vi "BNC555.Read Channel Parameters.vi"(0 "i ref in":refnum<vi>, 2 "Channel (1: Chan A)":i32(ring)=1 items=["System (To)", "Channel A", "Channel B", "Channel C", "Channel D", "Channel E", "Channel F", "Channel G", "Channel H"], 3 "Parameter":T1(ring), 5 "error in (no error)":errorcluster) -> (14 "i ref out":refnum<vi>, 19 "error out":errorcluster)   [LabVIEW 2014, in "BNC555.lvlib"]
doc: "This VI queries the connected channel state. The result is indicated as GUI element, parts are published as a dim service."
uses:
  BNC555.lvlib
  instr.lib/BNC555/BNC555 - Driver np.lvlib
  CSlibraries-extern/DimLVEvent/LVDimInterface/LVDimInterface.lvlib
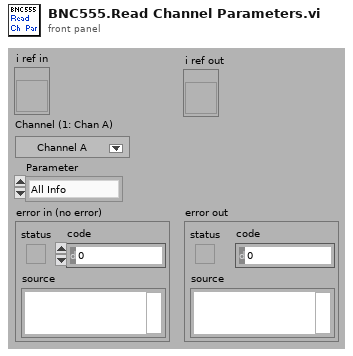
[diagram p1: front panel]
types:
  T1 = enum16{"All Info", "State (On/Off)", "Output Config", "Mode Config", "Pulse Config", "Gate Config"}
  T2 = typedef "BNC555.lvlib/BNC555.i attribute.ctl" = cluster{"Information":cluster{"VISA resource name":refnum<visa-resource-name>, "Baud Rate (1:9600)":u16}, "Channel Array":T3[], "System":T4, "GUI Refs":cluster{"Delete":refnum<vi>, "Information":refnum<vi>, "System":refnum<vi>, "Channel Array":refnum<vi>, "Device Error":refnum<vi>, "Instr Driver Revision":refnum<vi>, "Instr Firmware Revision":refnum<vi>, "Instr Option":refnum<vi>, "Self-Test Response":refnum<vi>}, "Service IDs Channelinfo":i32[], "Service ID T0 Mode":i32}
  T3 = typedef "BNC555 - Driver np.lvlib/BNC555 All Chan Parameters.ctl" = cluster{"Chan #":i32, "Chan State":bool, "Chan Delay":dbl, "Chan Width":dbl, "Chan Mode":enum16{"Normal", "Single", "Burst", "Divide by N"}, "Chan Burst #":u32, "Chan Divide #":u32, "Chan Pol Out":enum16{"Normal", "Complement", "Inverted"}, "Chan Level Out":enum16{"TTL", "Adjustable", "35 Volt"}, "Chan Lev Adjust":dbl, "Chan Gate Pol":enum16{"Normal", "Complement", "Inverted"}, "Chan Gate State":bool}
  T4 = typedef "BNC555 - Driver np.lvlib/BNC555 All Sys Parameters.ctl" = cluster{"Sys Period":dbl, "Sys Oscillator":bool, "Sys Mode":enum16{"Normal", "Single", "Burst", "Duty Cycle"}, "Sys Burst #":u32, "Sys DC On":u32, "Sys DC Off":u32, "Sys Trig Mode":enum16{"Disabled", "Triggered", "Gated"}, "Sys Trig Lev":dbl, "Sys Gate State":bool, "Sys Trig Edge":bool, "Sys State":bool}
  T5 = enum16{"All Info", "State (On/Off)", "Output Config", "Mode Config", "Pulse Config", "Gate Config"}[]
  T6 = enum16{"Normal", "Single", "Burst", "Divide by N"}
  T7 = typedef "BNC555 All Chan Parameters.ctl" = cluster{"Chan #":i32, "Chan State":bool, "Chan Delay":dbl, "Chan Width":dbl, "Chan Mode":enum16{"Normal", "Single", "Burst", "Divide by N"}, "Chan Burst #":u32, "Chan Divide #":u32, "Chan Pol Out":enum16{"Normal", "Complement", "Inverted"}, "Chan Level Out":enum16{"TTL", "Adjustable", "35 Volt"}, "Chan Lev Adjust":dbl, "Chan Gate Pol":enum16{"Normal", "Complement", "Inverted"}, "Chan Gate State":bool}
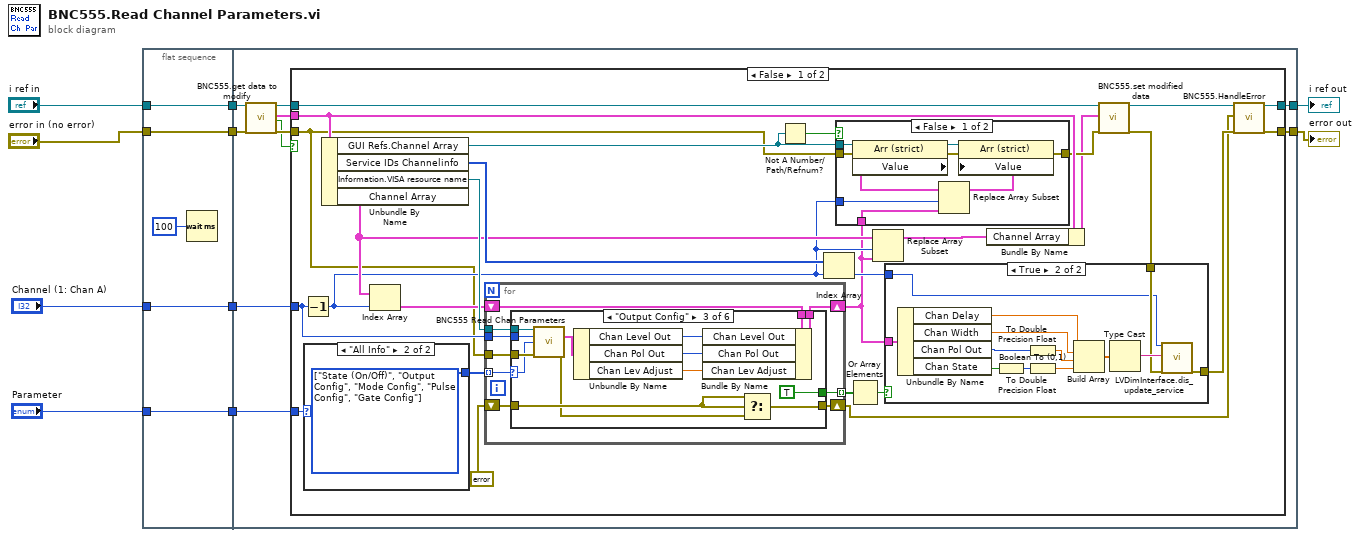
[diagram p0: block diagram]
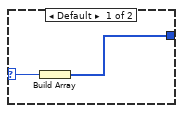
[diagram p2: hidden frame]
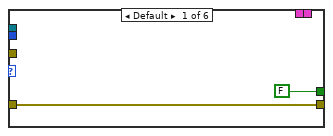
[diagram p4: hidden frame]
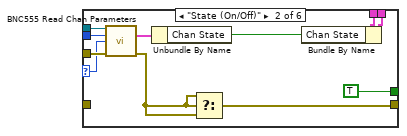
[diagram p5: hidden frame]
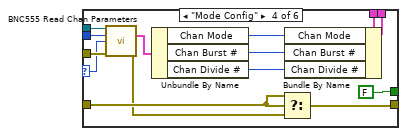
[diagram p6: hidden frame]
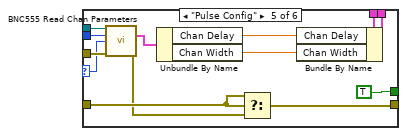
[diagram p7: hidden frame]
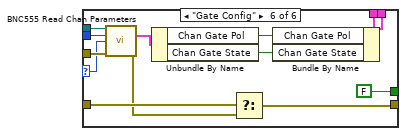
[diagram p8: hidden frame]
diagram:
  n1 = flat-sequence {
    tunnel: "Parameter" -> [w12]
    tunnel: "Channel (1: Chan A)" -> [w13]
    tunnel: "error in (no error)" -> [w14]
    tunnel: "i ref in" -> [w15]
    tunnel: [w15] -> w4
    tunnel: [w14] -> w3
    tunnel: [w13] -> w2
    tunnel: [w12] -> w1
    tunnel: [w19] -> w7
    tunnel: [w18] -> w6
    tunnel: w4 -> [w25]
    tunnel: w3 -> [w24]
    tunnel: w2 -> [w21]
    tunnel: w1 -> [w16]
    frame #0 {
      n2 = Wait (ms)(milliseconds to wait=u32 100) -> ()  [unwired: 1 out]
    }
    frame #1 {
      n3 = call "BNC555.get data to modify.vi"("i ref in"=w25, "error in (no error)"=w24) -> ("i ref out"=w22:refnum<vi>, "i attribute"=w23:T2, "timed out"=w17:bool, "error out"=w20:errorcluster)  [unwired: 14 in]
      n4 = case shown="False" w17 {
        tunnel: w23 -> [w49 _]
        tunnel: w22 -> [w40 w158]
        tunnel: w21 -> [w43 _]
        tunnel: w20 -> [w26 w157]
        tunnel: [w32 w157] -> w19
        tunnel: [w34 w158] -> w18
        tunnel: w16 -> [w27 _]
        frame False {
          n5 = Decrement(x=w43) -> (x-1=w37:i32)
          n6 = case shown="\"All Info\"" w27 {
            selector: w27 -> [w54 _]
            tunnel: [w53 w55] -> w44
            frame Default {
              n7 = Build Array(w54) -> (w53:T5)
            }
            frame "All Info" {
              w55 = T5 [enum."State (On/Off)", enum."Output Config", enum."Mode Config", enum."Pulse Config", enum."Gate Config"] items=["All Info", "State (On/Off)", "Output Config", "Mode Config", "Pulse Config", "Gate Config"]
            }
          }
          n8 = Unbundle By Name(w49) -> ("GUI Refs.Channel Array"=w47:refnum<vi>, "Service IDs Channelinfo"=w51:i32[], "Information.VISA resource name"=w46:refnum<visa-resource-name>, "Channel Array"=w41:T3[])
          n9 = Index Array(array=w41, index=w37) -> (element=w45:T3)
          n10 = for {
            shift-right: [w78] -> w30
            shift-left: w45 -> [w77]
            tunnel: w46 -> [w76]
            tunnel: w26 -> [w75]
            tunnel: w44 -> [w73] mode=indexing
            tunnel: w43 -> [w74]
            shift-right: [w72] -> w28
            shift-left: errorcluster {"status"=FALSE, "code"=0, "source"=""} ("error out") -> [w71]
            tunnel: [w70] -> w31 mode=indexing
            n11 = case shown="\"Output Config\"" w73 {
              selector: w73 -> [_ w86 w100 w114 w127 w140]
              tunnel: [w81 w92 w106 w120 w133 w146] -> w78
              tunnel: w77 -> [w81 w91 w105 w119 w132 w145]
              tunnel: w76 -> [_ w90 w104 w118 w131 w144]
              tunnel: w75 -> [_ w88 w102 w116 w129 w142]
              tunnel: w74 -> [_ w87 w101 w115 w128 w141]
              tunnel: [w80 w84 w99 w113 w126 w139] -> w72
              tunnel: w71 -> [w80 _ w98 w112 w125 w138]
              tunnel: [FALSE TRUE TRUE FALSE TRUE FALSE] -> w70
              frame Default {
              }
              frame "State (On/Off)" {
                n12 = call "BNC555 Read Chan Parameters.vi"("VISA resource"=w90, "Channel (1: Chan A)"=w87, "Parameter (1:State)"=w86, "error in (no error)"=w88) -> ("Channel Parameters"=w89:T3, "error out"=w82:errorcluster)  [unwired: 9 in, 1 out]
                n13 = Unbundle By Name(w89) -> ("Chan State"=w85:bool)
                n14 = Select(t=w82, s=w82, f=w82) -> (s? t:f=w84:errorcluster)
                n15 = Bundle By Name(cluster=w91, "Chan State"=w85) -> (w92:T3)
              }
              frame "Output Config" {
                n16 = call "BNC555 Read Chan Parameters.vi"("VISA resource"=w104, "Channel (1: Chan A)"=w101, "Parameter (1:State)"=w100, "error in (no error)"=w102) -> ("Channel Parameters"=w103:T3, "error out"=w95:errorcluster)  [unwired: 9 in, 1 out]
                n17 = Unbundle By Name(w103) -> ("Chan Level Out"=w97:enum16{"TTL", "Adjustable", "35 Volt"}, "Chan Pol Out"=w94:enum16{"Normal", "Complement", "Inverted"}, "Chan Lev Adjust"=w96:dbl)
                n18 = Bundle By Name(cluster=w105, "Chan Level Out"=w97, "Chan Pol Out"=w94, "Chan Lev Adjust"=w96) -> (w106:T3)
                n19 = Select(t=w98, s=w98, f=w95) -> (s? t:f=w99:errorcluster)
              }
              frame "Mode Config" {
                n20 = call "BNC555 Read Chan Parameters.vi"("VISA resource"=w118, "Channel (1: Chan A)"=w115, "Parameter (1:State)"=w114, "error in (no error)"=w116) -> ("Channel Parameters"=w117:T3, "error out"=w109:errorcluster)  [unwired: 9 in, 1 out]
                n21 = Unbundle By Name(w117) -> ("Chan Mode"=w111:T6, "Chan Burst #"=w108:u32, "Chan Divide #"=w110:u32)
                n22 = Select(t=w112, s=w112, f=w109) -> (s? t:f=w113:errorcluster)
                n23 = Bundle By Name(cluster=w119, "Chan Mode"=w111, "Chan Burst #"=w108, "Chan Divide #"=w110) -> (w120:T3)
              }
              frame "Pulse Config" {
                n24 = call "BNC555 Read Chan Parameters.vi"("VISA resource"=w131, "Channel (1: Chan A)"=w128, "Parameter (1:State)"=w127, "error in (no error)"=w129) -> ("Channel Parameters"=w130:T3, "error out"=w122:errorcluster)  [unwired: 9 in, 1 out]
                n25 = Unbundle By Name(w130) -> ("Chan Delay"=w123:dbl, "Chan Width"=w124:dbl)
                n26 = Select(t=w125, s=w125, f=w122) -> (s? t:f=w126:errorcluster)
                n27 = Bundle By Name(cluster=w132, "Chan Delay"=w123, "Chan Width"=w124) -> (w133:T3)
              }
              frame "Gate Config" {
                n28 = call "BNC555 Read Chan Parameters.vi"("VISA resource"=w144, "Channel (1: Chan A)"=w141, "Parameter (1:State)"=w140, "error in (no error)"=w142) -> ("Channel Parameters"=w143:T3, "error out"=w135:errorcluster)  [unwired: 9 in, 1 out]
                n29 = Unbundle By Name(w143) -> ("Chan Gate Pol"=w136:enum16{"Normal", "Complement", "Inverted"}, "Chan Gate State"=w137:bool)
                n30 = Select(t=w138, s=w138, f=w135) -> (s? t:f=w139:errorcluster)
                n31 = Bundle By Name(cluster=w145, "Chan Gate Pol"=w136, "Chan Gate State"=w137) -> (w146:T3)
              }
            }
          }
          n32 = Not A Number/Path/Refnum?(number/path/refnum=w47) -> (NaN/Path/Refnum?=w52:bool)
          n33 = Index Array(array=w51, index=w37) -> (element=w50:i32)
          n34 = case shown="False" w52 {
            tunnel: [w155 w156] -> w39
            tunnel: w26 -> [w150 w156]
            tunnel: w47 -> [w152 _]
            tunnel: w30 -> [w148 _]
            tunnel: w37 -> [w147 _]
            frame False {
              n35 = property class="Arr (strict)"(reference=w152, error in=w150) -> (reference out=w151:refnum<vi>, error out=w149:errorcluster, "Value"=w154:T7[])
              n36 = Replace Array Subset(array=w154, new element=w148, index=w147) -> (w153:T7[])
              n37 = property class="Arr (strict)"(reference=w151, error in=w149, "Value"=w153) -> (error out=w155:errorcluster)  [unwired: 1 out]
            }
            frame True {
            }
          }
          n38 = Or Array Elements(Boolean array=w31) -> (logical OR=w29:bool)
          n39 = Replace Array Subset(array=w41, new element=w30, index=w37) -> (w48:T3[])
          n40 = Bundle By Name(cluster=w49, "Channel Array"=w48) -> (w38:T2)
          n41 = call "BNC555.set modified data.vi"("i ref in"=w40, "i attribute"=w38, "error in (no error)"=w39) -> ("i ref out"=w35:refnum<vi>, "error out"=w33:errorcluster)  [unwired: 15 in]
          n42 = case shown="True" w29 {
            tunnel: w50 -> [_ w57]
            tunnel: [w56 w67] -> w36
            tunnel: w33 -> [w56 w66]
            tunnel: w30 -> [_ w65]
            frame False {
            }
            frame True {
              n43 = Unbundle By Name(w65) -> ("Chan Delay"=w58:dbl, "Chan Width"=w59:dbl, "Chan Pol Out"=w64:enum16{"Normal", "Complement", "Inverted"}, "Chan State"=w62:bool)
              n44 = Boolean To (0,1)(Boolean=w62) -> (0, 1=w63:i16)
              n45 = To Double Precision Float(number=w64) -> (double precision float=w60:dbl)
              n46 = To Double Precision Float(number=w63) -> (double precision float=w61:dbl)
              n47 = Build Array(w58, w59, w60, w61) -> (w68:dbl[])
              n48 = Type Cast(x=w68) -> (*(type *) &x=w69:string)  [unwired: 1 in]
              n49 = call "LVDimInterface.dis_update_service.vi"("my_serviceID"=w57, "data"=w69, "error in (no error)"=w66) -> ("error out"=w67:errorcluster)  [unwired: 14 in, 2 out]
            }
          }
          n50 = call "BNC555.HandleError.vi"("i ref in"=w35, "Device error"=w28, "error in (no error)"=w36) -> ("i ref out"=w34:refnum<vi>, "error out"=w32:errorcluster)  [unwired: 15 in]
        }
        frame True {
        }
      }
    }
  }
  "i ref out" <- w6
  "error out" <- w7
